vi "Calculate INL.vi"(0 "Actual X":dbl[](array[numeric]), 1 "Best Fit?":bool, 5 "Actual Y":dbl[](array[numeric]), 7 "Ideal X":dbl[](array[numeric]), 9 "Ideal Y":dbl[](array[numeric]), 11 "Error in":errorcluster, 12 "ADC?":bool) -> (4 "INL X Plot values":dbl[](array[numeric]), 6 "INL Y Plot Values":dbl[](array[numeric]), 8 "INL Result values":dbl[](array[numeric]), 15 "Error out":errorcluster)   [LabVIEW 2020, in "INL DNL Test.lvclass"]
doc: "Calculates INL result based on bestfit/endpoint method"
uses:
  INL DNL Test.lvclass
  <vilib>/Analysis/6fits.llb/Curve Fitting Criteria.ctl
  <vilib>/Analysis/NI_AALPro.lvlib
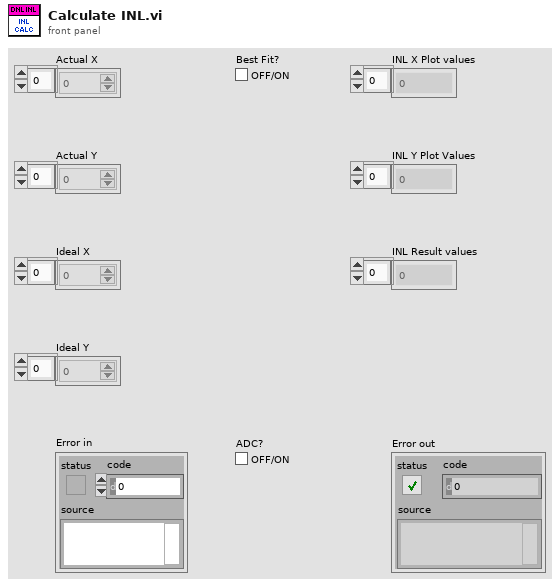
[diagram p1: front panel]
types:
  T1 = typedef "NI_AALPro.lvlib/Curve Fitting Criteria.ctl" = u16
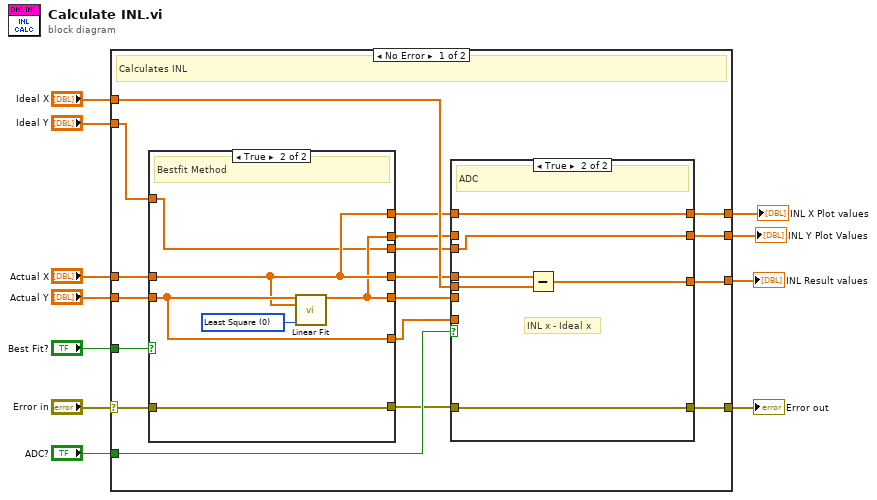
[diagram p0: block diagram]
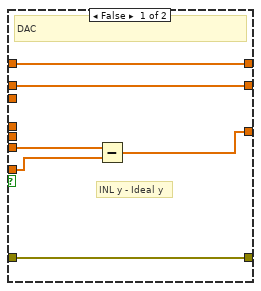
[diagram p3: hidden frame]
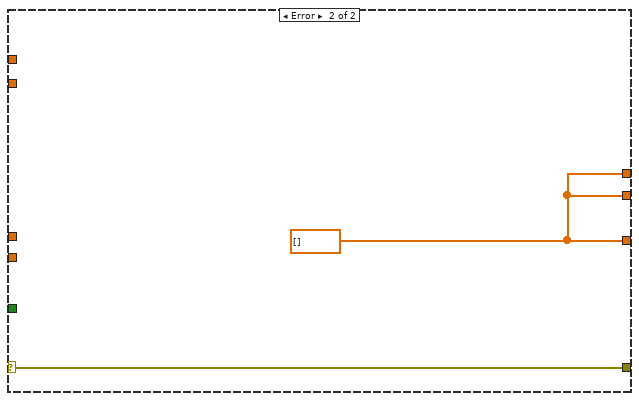
[diagram p4: hidden frame]
diagram:
  n1 = case shown="No Error" "Error in" {
    selector: "Error in" -> [w26 w53]
    tunnel: "Best Fit?" -> [w29 _]
    tunnel: "Actual X" -> [w28 _]
    tunnel: "Actual Y" -> [w27 _]
    tunnel: "Ideal X" -> [w24 _]
    tunnel: "Ideal Y" -> [w13 _]
    tunnel: "ADC?" -> [w25 _]
    tunnel: [w21 w53] -> w3
    tunnel: [w20 w52] -> w4
    tunnel: [w17 w52] -> w2
    tunnel: [w14 w52] -> w1
    frame No Error {
      # "Calculates INL"
      n2 = case shown="True" w29 {
        tunnel: w28 -> [w31 w36]
        tunnel: w27 -> [w30 w37]
        tunnel: [w30 w35] -> w18
        tunnel: [w31 w36] -> w23
        tunnel: w26 -> [w33 w38]
        tunnel: [w33 w38] -> w22
        tunnel: [w32 w37] -> w19
        tunnel: w13 -> [w32 w34]
        tunnel: [w31 w36] -> w16
        tunnel: [w30 w35] -> w15
        tunnel: [w30 w34] -> w12
        frame False {
          # "Endpoint Method"
        }
        frame True {
          w39 = T1 0 items=["Least Square", "Least Absolute Residual", "Bisquare"] ("method")
          # "Bestfit Method"
          n3 = call <vilib>:"Linear Fit.vi"("Y"=w37, "X"=w36, "method"=w39) -> ("Best Linear Fit"=w35:dbl[])  [unwired: 8 in, 4 out]
        }
      }
      n4 = case shown="True" w25 {
        tunnel: w24 -> [_ w49]
        tunnel: w23 -> [_ w50]
        tunnel: [w44 w51] -> w20
        tunnel: w18 -> [w45 _]
        tunnel: w22 -> [w43 w48]
        tunnel: [w43 w48] -> w21
        tunnel: w19 -> [w42 _]
        tunnel: w15 -> [w41 _]
        tunnel: [w41 w46] -> w17
        tunnel: w16 -> [w40 w47]
        tunnel: [w40 w47] -> w14
        tunnel: w12 -> [_ w46]
        frame False {
          # "INL y - Ideal y"
          # "DAC"
          n5 = Subtract(x=w45, y=w42) -> (x-y=w44:dbl[])
        }
        frame True {
          # "INL x - Ideal x"
          # "ADC"
          n6 = Subtract(x=w50, y=w49) -> (x-y=w51:dbl[])
        }
      }
    }
    frame Error {
      w52 = dbl[] []
    }
  }
  "INL Result values" <- w4
  "Error out" <- w3
  "INL Y Plot Values" <- w2
  "INL X Plot values" <- w1
